vi "configure assembly.vi"(8 "error in":errorcluster, 10 "assembly definition in":T2={"name"="", "Instance ID"=100, "Type"=enum."Producing", "Size (bytes)"=32, "big endian?"=FALSE}, 11 "EthernetIP configuration":refnum<class "EthernetIP configuration.lvclass">) -> (0 "error out":errorcluster, 1 "success":bool, 2 "assembly definition out":T2={"name"="", "Instance ID"=100, "Type"=enum."Producing", "Size (bytes)"=32, "big endian?"=FALSE}, 5 "changed":bool)   [LabVIEW 2013, in "EthernetIP editor node.lvclass"]
uses:
  EthernetIP editor node.lvclass
  <vilib>/NI/TBM Modules/Ethernet IP/configuration/EthernetIP configuration.lvclass
  <vilib>/NI/TBM Modules/Ethernet IP/configuration/assembly definition.ctl
  <vilib>/NI/TBM Modules/Ethernet IP/configuration/assembly type.ctl
  <vilib>/NI/TBM Modules/Ethernet IP/configuration/EthernetIP configuration.lvclass/EthernetIP configuration.ctl
  <vilib>/NI/TBM Modules/Ethernet IP/configuration/Read assemblies.vi
panel:
  in  "byte order":enum32{"Little", "Big"}(radio)
  in  "Size (bytes)":u32
  in  "Instance ID":u32
  in  "Asm Type":T1
  in  "Assembly Name (opt)":string
  in  "cancel":bool
  in  "ok":bool
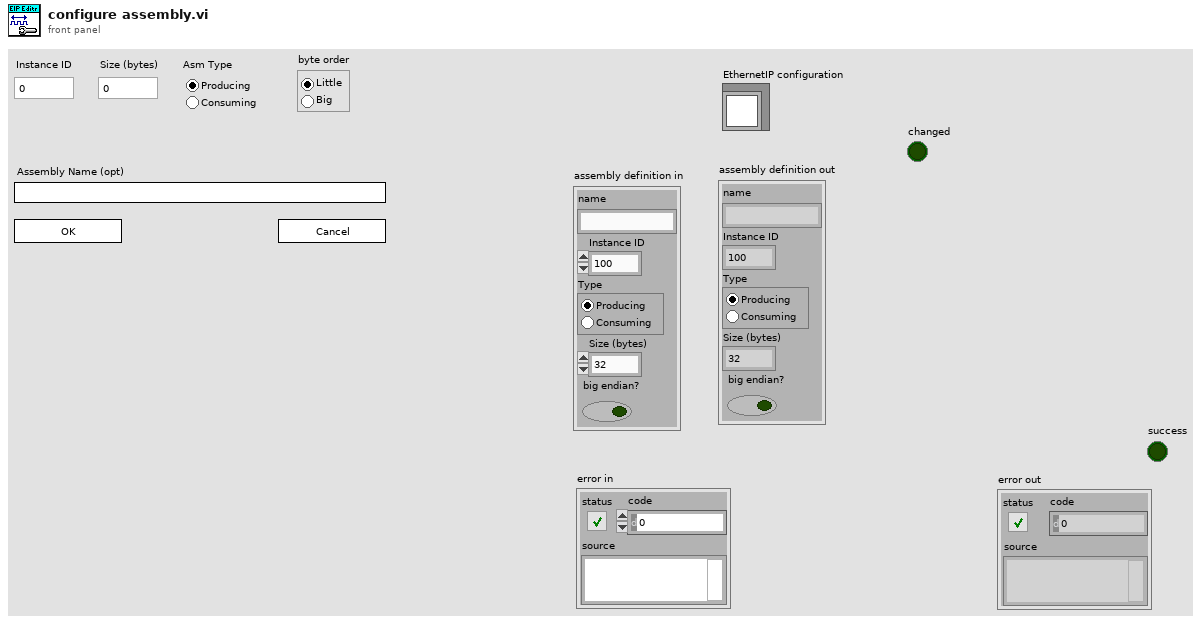
[diagram p1: front panel]
types:
  T1 = typedef "EthernetIP configuration.lvclass/assembly type.ctl" = enum32{"Producing", "Consuming"}
  T2 = typedef "EthernetIP configuration.lvclass/assembly definition.ctl" = cluster{"name":string, "Instance ID":u32, "Type":T1, "Size (bytes)":u32, "big endian?":bool}
  T3 = enum32{"Invalid", "Standard", "Closed", "Hidden", "Minimized", "Maximized"}
  T4 = enum32{"Invalid", "Default", "Floating", "Floating/Auto-Hide", "Modal"}
  T5 = enum32{"invalid app kind", "Development System", "Run Time System", "Student Edition", "Embedded LabVIEW", "Evaluation", "Custom"}
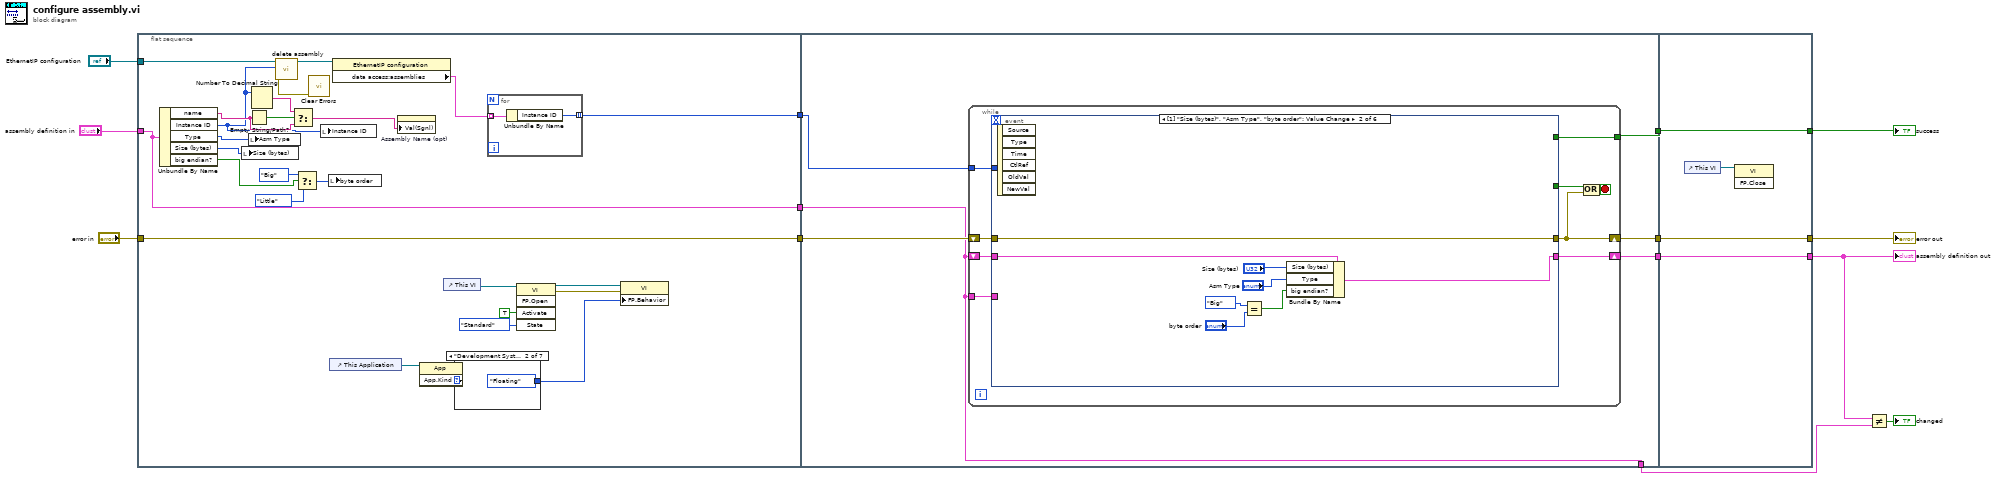
[diagram p0: block diagram]
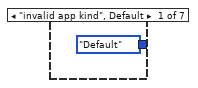
[diagram p2: hidden frame]
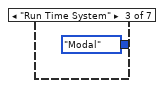
[diagram p3: hidden frame]
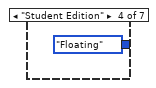
[diagram p4: hidden frame]
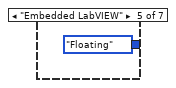
[diagram p5: hidden frame]
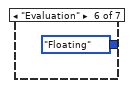
[diagram p6: hidden frame]
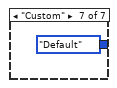
[diagram p7: hidden frame]
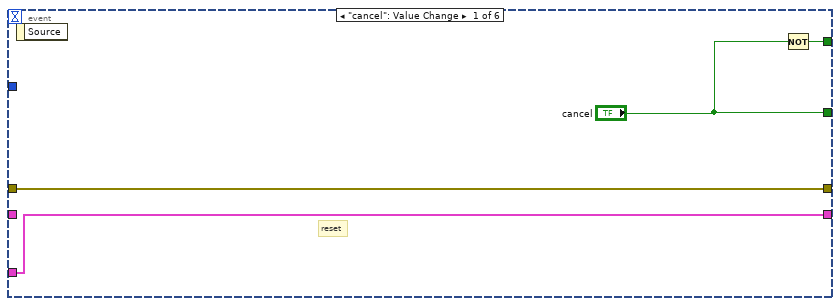
[diagram p8: hidden frame]
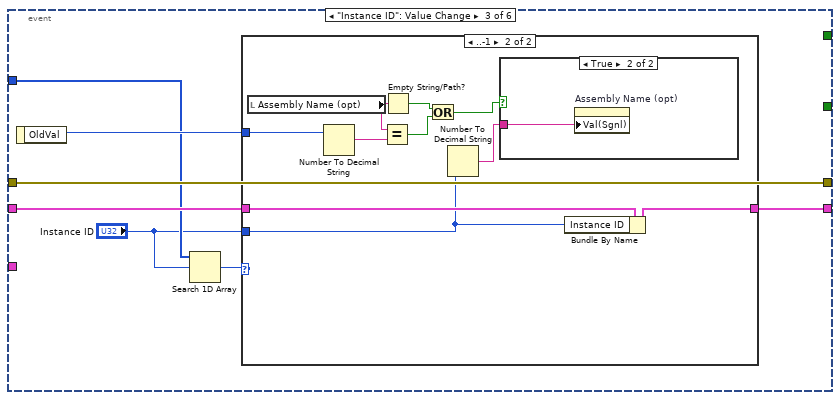
[diagram p9: hidden frame]
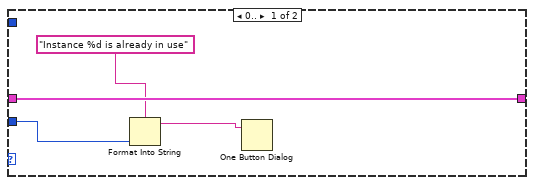
[diagram p10: hidden frame]
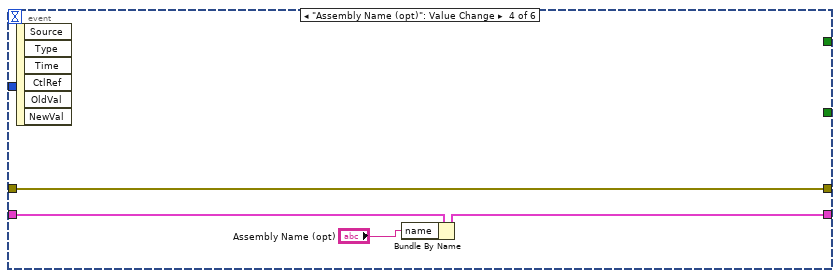
[diagram p12: hidden frame]
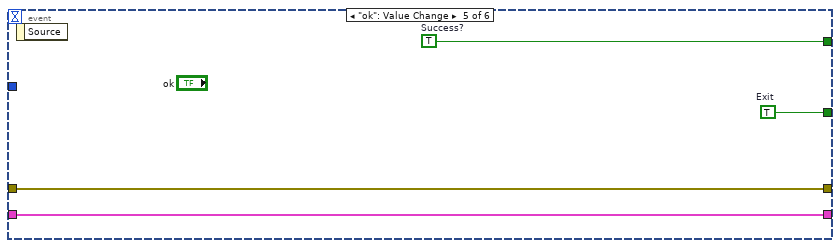
[diagram p13: hidden frame]
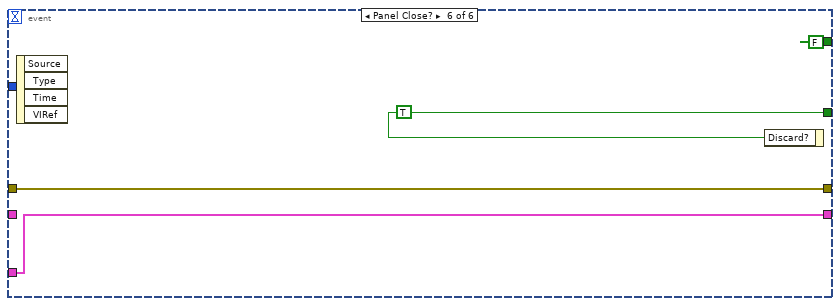
[diagram p14: hidden frame]
diagram:
  n1 = flat-sequence {
    tunnel: "error in" -> [w24]
    tunnel: "EthernetIP configuration" -> [w32]
    tunnel: "assembly definition in" -> [w20]
    tunnel: [w28] -> w5
    tunnel: [w24] -> w4
    tunnel: [w20] -> w3
    tunnel: [w55] -> w10
    tunnel: [w54] -> w9
    tunnel: [w53] -> w8
    tunnel: w5 -> [w50]
    tunnel: w4 -> [w52]
    tunnel: w3 -> [w51]
    tunnel: [w51] -> w2
    tunnel: [w112] -> w1
    tunnel: [w113] -> w12
    tunnel: [w114] -> w13
    tunnel: w10 -> [w114]
    tunnel: w9 -> [w113]
    tunnel: w8 -> [w112]
    frame #0 {
      n2 = Unbundle By Name(w20) -> ("name"=w26:string, "Instance ID"=w22:u32, "Type"=w23:T1, "Size (bytes)"=w21:u32, "big endian?"=w15:bool)
      n3 = local write "Size (bytes)"(w21) -> ()
      n4 = local write "Asm Type"(w23) -> ()
      n5 = Empty String/Path?(string/path=w26) -> (empty?=w27:bool)
      n6 = Number To Decimal String(number=w22) -> (decimal integer string=w25:string)  [unwired: 1 in]
      n7 = call <vilib>:"delete assembly.vi"("instance ID"=w22, "EthernetIP configuration in"=w32) -> ("error out"=w29:errorcluster, "EthernetIP configuration out"=w30:refnum<class "EthernetIP configuration.lvclass">)  [unwired: 7 in, 1 out]
      n8 = Select(t=w25, s=w27, f=w26) -> (s? t:f=w19:string)
      n9 = Select(t=enum32{"Little", "Big"}."Big" ("byte order"), s=w15, f=enum32{"Little", "Big"}."Little" ("byte order")) -> (s? t:f=w16:enum32{"Little", "Big"})
      n10 = call <vilib>:"Clear Errors.vi"("error in (no error)"=w29) -> ()  [unwired: 6 in, 1 out]
      n11 = local write "Instance ID"(w22) -> ()
      n12 = local write "byte order"(w16) -> ()
      n13 = control-ref of="This Application"() -> (w35:refnum<vi>)
      n14 = property class="EthernetIP configuration"(reference=w30) -> ("data access:assemblies"=w31:T2[])  [unwired: 1 in, 2 out]
      n15 = property on="Assembly Name (opt)" class="Str"("Val(Sgnl)"=w19) -> ()  [unwired: 2 in, 2 out]
      n16 = property class="App"(reference=w35) -> ("App.Kind"=w34:T5)  [unwired: 1 in, 2 out]
      n17 = control-ref of="This VI"() -> (w36:refnum<vi>)
      n18 = case shown="\"Development System\"" w34 {
        tunnel: [T4."Default" ("Front Panel Window:Behavior") T4."Floating" ("Front Panel Window:Behavior") T4."Modal" ("Front Panel Window:Behavior") T4."Floating" ("Front Panel Window:Behavior") T4."Floating" ("Front Panel Window:Behavior") T4."Floating" ("Front Panel Window:Behavior") T4."Default" ("Front Panel Window:Behavior")] -> w33
        frame "invalid app kind", Default {
        }
        frame "Development System" {
        }
        frame "Run Time System" {
        }
        frame "Student Edition" {
        }
        frame "Embedded LabVIEW" {
        }
        frame "Evaluation" {
        }
        frame "Custom" {
        }
      }
      n19 = for {
        tunnel: w31 -> [w42] mode=indexing
        tunnel: [w41] -> w28 mode=indexing
        n20 = Unbundle By Name(w42) -> ("Instance ID"=w41:u32)
      }
      n21 = invoke class="VI" method="FP.Open"(reference=w36, "Activate"=TRUE ("Activate?"), "State"=T3."Standard") -> (reference out=w39:refnum<vi>, error out=w40:errorcluster)  [unwired: 2 in, 3 out]
      n22 = property class="VI"(reference=w39, error in=w40, "FP.Behavior"=w33) -> ()  [unwired: 2 out]
    }
    frame #1 {
      n23 = while {
        shift-right: [w59] -> w54
        shift-left: w52 -> [w64]
        tunnel: [w63] -> w55
        shift-right: [w57] -> w53
        shift-left: w51 -> [w60]
        tunnel: w51 -> [w58]
        tunnel: w50 -> [w56]
        stop <- w61 stop-if-true
        n24 = event shown="[1] \"Size (bytes)\", \"Asm Type\", \"byte order\": Value Change" {
          selector: _ -> [_ _ _ _ _ _]
          dyn-events: _ -> [_ _ _ _ _ _]
          timeout: _ -> [_ _ _ _ _ _]
          tunnel: w64 -> [w68 w76 w83 w102 w106 w110]
          tunnel: [w68 w76 w83 w102 w106 w110] -> w59
          tunnel: [w67 _ _ _ w103 FALSE] -> w63
          tunnel: ["cancel" _ _ _ w104 w108] -> w62
          tunnel: w60 -> [_ w75 w82 w101 w105 _]
          tunnel: [w65 w74 w81 w100 w105 w107] -> w57
          tunnel: w58 -> [w65 _ _ _ _ w107]
          tunnel: w56 -> [_ _ w79 _ _ _]
          event "cancel": Value Change {
            # "reset"
            n25 = event-data() -> ()  [unwired: 1 in, 1 out]
            n26 = Not(x="cancel") -> (.not. x?=w67:bool)
          }
          event "Size (bytes)", "byte order": Value Change {
            n27 = event-data() -> ()  [unwired: 1 in, 6 out]
            n28 = Equal?(x=enum32{"Little", "Big"}."Big" ("byte order"), y="byte order") -> (x = y?=w69:bool)
            n29 = Bundle By Name(cluster=w75, "Size (bytes)"="Size (bytes)", "Type"="Asm Type", "big endian?"=w69) -> (w74:T2)
          }
          event "Instance ID": Value Change {
            n30 = event-data() -> ("OldVal"=w80:u32)  [unwired: 1 in]
            n31 = Search 1D Array(1D array=w79, element="Instance ID") -> (index of element=w77:i32)  [unwired: 1 in]
            n32 = case shown="..-1" w77 {
              tunnel: w82 -> [w87 w97]
              tunnel: [w87 w96] -> w81
              tunnel: w80 -> [_ w95]
              tunnel: "Instance ID" -> [w86 w88]
              frame 0.. {
                n33 = Format Into String(format string="Instance %d is already in use", w86) -> (resulting string=w85:string)  [unwired: 2 in, 1 out]
                n34 = One Button Dialog(message=w85) -> ()  [unwired: 1 in, 1 out]
              }
              frame ..-1 {
                n35 = local read "Assembly Name (opt)"() -> (w91:string)
                n36 = Number To Decimal String(number=w95) -> (decimal integer string=w92:string)  [unwired: 1 in]
                n37 = Equal?(x=w91, y=w92) -> (x = y?=w93:bool)
                n38 = Empty String/Path?(string/path=w91) -> (empty?=w94:bool)
                n39 = Or(x=w94, y=w93) -> (x .or. y?=w90:bool)
                n40 = Number To Decimal String(number=w88) -> (decimal integer string=w89:string)  [unwired: 1 in]
                n41 = case shown="True" w90 {
                  tunnel: w89 -> [_ w98]
                  frame False {
                  }
                  frame True {
                    n42 = property on="Assembly Name (opt)" class="Str"("Val(Sgnl)"=w98) -> ()  [unwired: 2 in, 2 out]
                  }
                }
                n43 = Bundle By Name(cluster=w97, "Instance ID"=w88) -> (w96:T2)
              }
            }
          }
          event "Assembly Name (opt)": Value Change {
            n44 = event-data() -> ()  [unwired: 1 in, 6 out]
            n45 = Bundle By Name(cluster=w101, "name"="Assembly Name (opt)") -> (w100:T2)
          }
          event "ok": Value Change {
            w103 = TRUE  # Success?
            w104 = TRUE  # Exit
            n46 = event-data() -> ()  [unwired: 1 in, 1 out]
          }
          event Panel Close? {
            w108 = TRUE ("cancel")
            n47 = event-data() -> ()  [unwired: 1 in, 4 out]
            n48 = event-data("Discard?"=w108) -> ()  [unwired: 1 in, 1 out]
          }
        }
        n49 = Compound Arithmetic op=OR(w62, w59) -> (w61:bool)
      }
    }
    frame #2 {
      n50 = control-ref of="This VI"() -> (w111:refnum<vi>)
      n51 = invoke class="VI" method="FP.Close"(reference=w111) -> ()  [unwired: 2 in, 3 out]
    }
  }
  n52 = Not Equal?(x=w1, y=w2) -> (x != y?=→"changed":bool)
  "error out" <- w12
  "success" <- w13
  "assembly definition out" <- w1
